vi "TDC_deInit.vi"(8 "Error In":errorcluster) -> (0 "Error Out":errorcluster)   [LabVIEW 2013]
uses:
  lib/tdcbase.dll
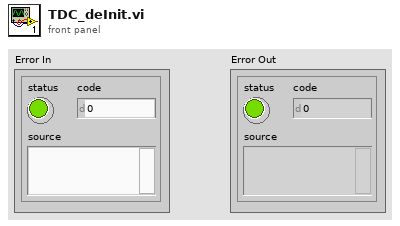
[diagram p1: front panel]
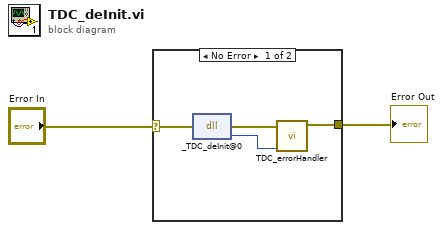
[diagram p0: block diagram]
diagram:
  n1 = case shown="No Error" "Error In" {
    selector: "Error In" -> [w6 w7]
    tunnel: [w4 w7] -> w1
    frame No Error {
      n2 = dll-call lib="C:/Users/science/Desktop/NVExperimeent/Labview/QUTAU-15_06_25/userlib/lib/tdcbase.dll" fn="_TDC_deInit@0"(error in=w6) -> (error out=w5:errorcluster, "return type"=w3:i32)  [unwired: 2 in, 1 out]
      n3 = call "TDC_errorHandler.vi"("quTAU Return Code"=w3, "Error In"=w5) -> ("Error Out"=w4:errorcluster)  [unwired: 9 in]
    }
    frame Error {
    }
  }
  "Error Out" <- w1
